vi "Read UID.vi"(8 "error in":errorcluster, 11 "CEF_Configuration in":refnum<class "CEF_serializable configuration.lvclass">) -> (0 "error out":errorcluster, 2 "instance id":string, 3 "CEF_Configuration out":refnum<class "CEF_serializable configuration.lvclass">)   [LabVIEW 2023, in "CEF.lvlib" / "CEF_serializable configuration.lvclass"]
doc: "Provides the instance name of a given configuration/runtime class pairing. This instance may be used as an identifier to differentiate between configurations. On first call, this instance ID is generated.Copyright 2017 National Instruments Corporation\n\nLicensed under the Apache License, Version 2.0 (the \"License\"); you may not use this file except in compliance with the License. You may obtain a copy of the License at http://www.apache.org/licenses/LICENSE-2.0\nUnless required by applicable law or agreed to in writing, software distributed under the License is distributed on an \"AS IS\" BASIS, WITHOUT WARRANTIES OR CONDITIONS OF ANY KIND, either express or implied. See the License for the specific language governing permissions and limitations under the License."
uses:
  CEF_serializable configuration.lvclass
  CEF_serializable configuration.lvclass/CEF_serializable configuration.ctl
  CEF.lvlib
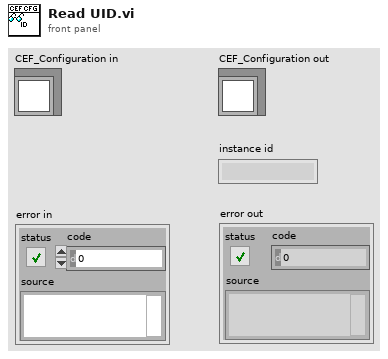
[diagram p1: front panel]
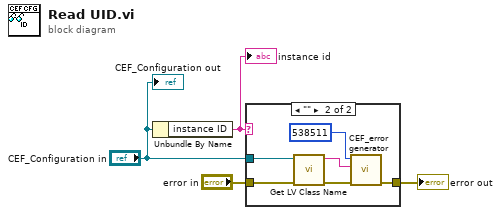
[diagram p0: block diagram]
diagram:
  n1 = Unbundle By Name("CEF_Configuration in") -> ("instance ID"=w2:string)
  "instance id" <- w2
  n2 = case shown="\"\"" w2 {
    tunnel: [w5 w10] -> w4
    tunnel: "error in" -> [w5 w11]
    tunnel: "CEF_Configuration in" -> [_ w6]
    frame Default {
    }
    frame "" {
      n3 = call <vilib>:"Get LV Class Name.vi"("error in (no error)"=w11, "object"=w6) -> ("error out"=w8:errorcluster, "class name"=w7:string)  [unwired: 8 in]
      n4 = call "CEF_error generator.vi"("error in"=w8, "append error message"=w7, "error code (0)"=538511) -> ("error out"=w10:errorcluster)  [unwired: 6 in]
    }
  }
  "error out" <- w4
  "CEF_Configuration out" <- "CEF_Configuration in"
